vi "Test-exit.vi"(8 "error in (no error)":errorcluster, 11 "ModComm in":T1) -> (0 "error out":errorcluster, 1 "Exit?":bool, 3 "ModComm out":T1)   [LabVIEW 2013, in "Server.lvlib" / "Server.lvclass"]
uses:
  Server.lvclass
  Object-reference.ctl
  Server.lvclass/Server.ctl
  Read Exit.vi
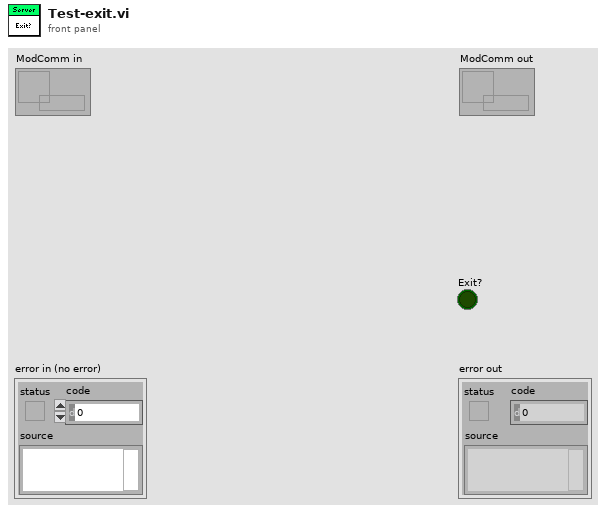
[diagram p1: front panel]
types:
  T1 = typedef "Server.lvlib/Server.lvclass/Object-reference.ctl" = refnum<data-value>
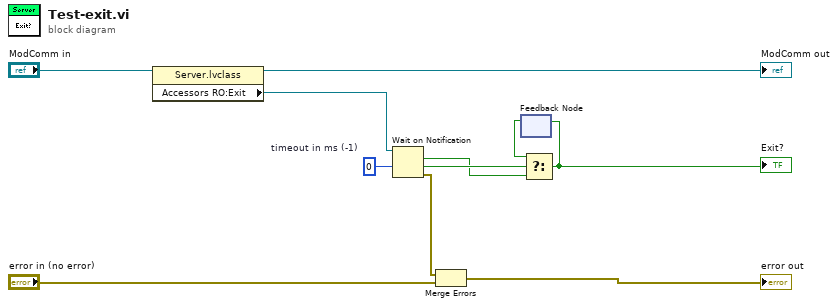
[diagram p0: block diagram]
diagram:
  w7 = 0  # timeout in ms (-1)
  n1 = property class="Server.lvclass"(reference="ModComm in") -> (reference out=→"ModComm out":T1, "Accessors RO:Exit"=w6:refnum<notifier>)  [unwired: 1 in, 1 out]
  n2 = Wait on Notification(notifier=w6, timeout in ms (-1)=w7) -> (notification=w3:bool, timed out?=w5:bool, error out=w11:errorcluster)  [unwired: 2 in, 1 out]
  n3 = Merge Errors(w11, "error in (no error)") -> (→"error out":errorcluster)
  n4 = feedback #1() -> (w4:bool)  [unwired: 1 in]
  n5 = Select(t=w4, s=w5, f=w3) -> (s? t:f=w8:bool)
  "Exit?" <- w8
  n6 = feedback-in #1(w8) -> ()
